vi "calcRampPressureOutputSTRamp.vi"(8 "error in (no error)":errorcluster, 11 "Model in":refnum<class "Model.lvclass">) -> (0 "error out":errorcluster, 3 "Model out":refnum<class "Model.lvclass">)   [LabVIEW 2015, in "Model.lvclass"]
uses:
  Model.lvclass
  Model.lvclass/Model.ctl
  <userlib>/Common/Devices/PressureValve/PressureValve/PressureValve.lvclass/PressureValve.ctl
  <userlib>/Common/ILC/ILC/ILC.lvclass/ILC.ctl
  <userlib>/Common/ILC/ILC/ILC.lvclass
  <userlib>/Common/Devices/PressureValve/PressureValve/PressureValve.lvclass
  ApplicationElements/SystemController/SystemController.lvclass
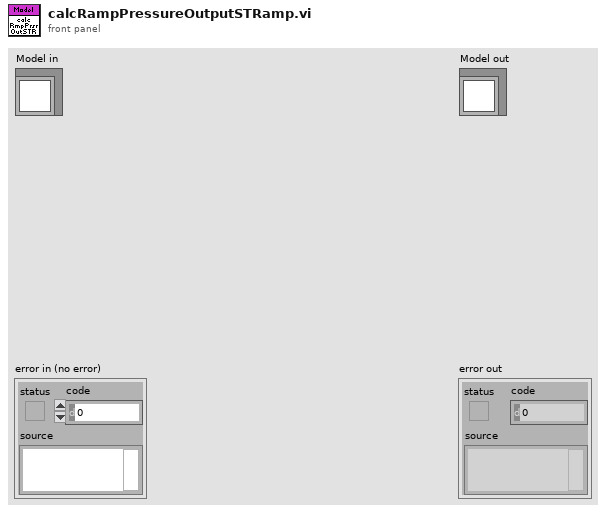
[diagram p1: front panel]
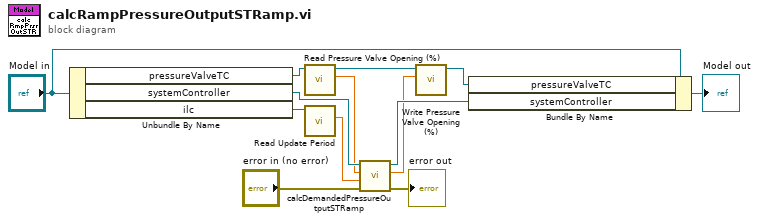
[diagram p0: block diagram]
diagram:
  n1 = Unbundle By Name("Model in") -> ("pressureValveTC"=w3:refnum<class "PressureValveTC.lvclass">, "systemController"=w9:refnum<class "SystemController.lvclass">, "ilc"=w7:refnum<class "ILC.lvclass">)
  n2 = call <userlib>:"Read Pressure Valve Opening (%).vi"("PressureValve in"=w3) -> ("Pressure Valve Opening (%)"=w1:dbl, "PressureValve out"=w2:refnum<class "PressureValveTC.lvclass">)  [unwired: 9 in]
  n3 = call <userlib>:"Read Update Period.vi"("ILC in"=w7) -> ("Update Period"=w6:dbl[unit])  [unwired: 9 in, 1 out]
  n4 = call "calcDemandedPressureOutputSTRamp.vi"("error in (no error)"="error in (no error)", "loopPeriod"=w6, "Pressure Valve Opening (%)"=w1, "SystemController in"=w9) -> ("error out"=→"error out":errorcluster, "rampOutput (%)"=w5:dbl, "SystemController out"=w8:refnum<class "SystemController.lvclass">)  [unwired: 5 in]
  n5 = call <userlib>:"Write Pressure Valve Opening (%).vi"("Pressure Valve Opening (%)"=w5, "PressureValve in"=w2) -> ("PressureValve out"=w4:refnum<class "PressureValveTC.lvclass">)  [unwired: 9 in]
  n6 = Bundle By Name(cluster="Model in", "pressureValveTC"=w4, "systemController"=w8) -> (→"Model out":refnum<class "Model.lvclass">)
